vi "U16 to U8H and U8L.vi"(4 "U16":u16) -> (0 "Lower Byte":u8 caption="低字节", 1 "Higher Byte":u8 caption="高字节")   [LabVIEW 2023, in "Longer Pump dLSP501 Series.lvlib"]
uses:
  <instrlib>/Longer Pump dLSP501 Modbus RTU Series/Longer Pump dLSP501 Series.lvlib
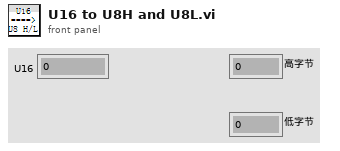
[diagram p1: front panel]
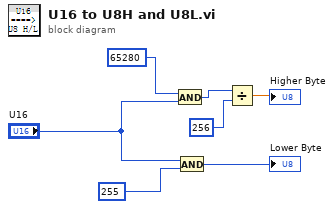
[diagram p0: block diagram]
diagram:
  n1 = And(x=u16 65280, y="U16") -> (x .and. y?=w2:u16)
  n2 = And(x="U16", y=u16 255) -> (x .and. y?=→"Lower Byte":u16)
  n3 = Divide(x=w2, y=256) -> (x/y=→"Higher Byte":dbl)
